vi "Log Data to File.vi"(8 "error in (no error)":errorcluster, 10 "Data to log":waveform(dbl)[](array[waveform]), 11 "TDMS File Reference":refnum<k34>) -> (0 "error out":errorcluster)   [LabVIEW 2019, in "Logger.lvlib"]
doc: "This VI uses the TDMS Write function to write data to a TDMS file.\n_____\nBased on Delacor QMH Project Template 5.0.0.82."
uses:
  Logger.lvlib
  <vilib>/Utility/file.llb/Write Delimited Spreadsheet (DBL).vi
panel:
  out "TDMS File Reference, not used":refnum<k34>
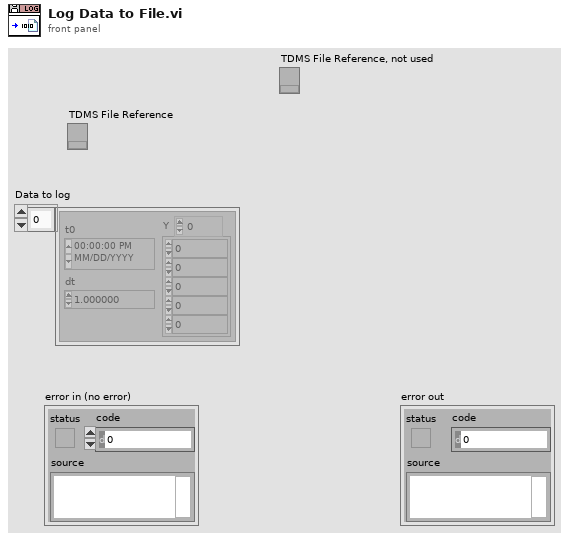
[diagram p1: front panel]
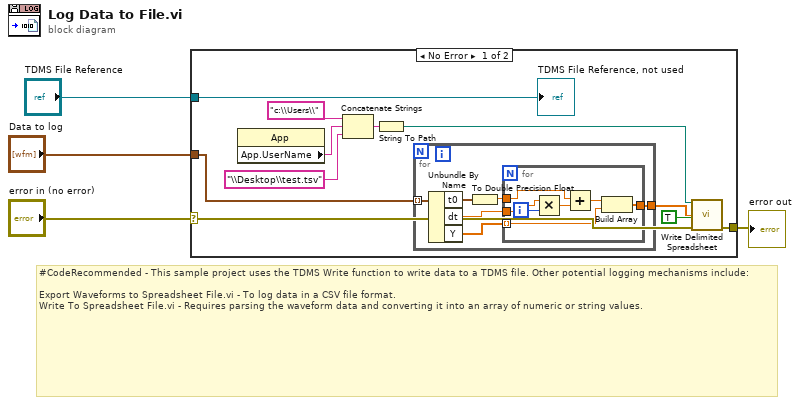
[diagram p0: block diagram]
diagram:
  # "#CodeRecommended - This sample project uses the TDMS Write function to write data to a TDMS file. Other potential logging mechanisms include:\n\nExport Waveforms to Spreadsheet File.vi - To log data in a CSV file format.\nWrite To Spreadsheet File.vi - Requires parsing the waveform data and converting it into an array of numeric or string values."
  n1 = case shown="No Error" "error in (no error)" {
    selector: "error in (no error)" -> [w8 w29]
    tunnel: "Data to log" -> [w10 _]
    tunnel: [w7 w29] -> w3
    tunnel: "TDMS File Reference" -> [w15 _]
    frame No Error {
      n2 = property class="App"() -> ("App.UserName"=w13:string)  [unwired: 2 in, 2 out]
      n3 = Concatenate Strings("c:\\Users\\", w13, "\\Desktop\\test.tsv") -> (w11:string)
      n4 = String To Path(string=w11) -> (path=w6:path)
      n5 = for {
        tunnel: w10 -> [w21] mode=indexing
        tunnel: [w19] -> w5
        n6 = Unbundle By Name(w21) -> ("t0"=w17:timestamp, "dt"=w20:dbl, "Y"=w18:dbl[])
        n7 = To Double Precision Float(number=w17) -> (double precision float=w16:dbl)
        n8 = for {
          tunnel: w20 -> [w27]
          tunnel: [w25] -> w19
          tunnel: w18 -> [w23] mode=indexing
          tunnel: w16 -> [w24]
          i -> [w28]
          n9 = Multiply(x=w27, y=w28) -> (x*y=w26:dbl)
          n10 = Add(x=w24, y=w26) -> (x+y=w22:dbl)
          n11 = Build Array(w22, w23) -> (w25:dbl[])
        }
      }
      n12 = call-poly <vilib>:"Write Delimited Spreadsheet.vi"("file path (dialog if empty)"=w6, "1D data"=w5, "append to file? (new file:F)"=TRUE, "error in (no error)"=w8) -> ("error out"=w7:errorcluster)  [unwired: 10 in, 1 out]
      "TDMS File Reference, not used" <- w15
    }
    frame Error {
    }
  }
  "error out" <- w3
